vi "Vin_Vout_2015.vi"(2 "V in volt":dbl format="%0.2f", 3 "Fondo Scala 6024":dbl(ring)=10.0 items=["10"=10.0, "5"=5.0, "0.5"=0.5, "0.05"=0.05], 4 "Canale Ingresso":tag="Dev1/ai0", 5 "Canale uscita":tag="Dev1/ao0") -> (0 "standard deviation":dbl format="%.5f", 1 "mean Vout":dbl format="%.5f")   [LabVIEW 2014]
uses:
  <vilib>/DAQmx/write.llb/DAQmx Write (Analog DBL 1Chan 1Samp).vi
  <vilib>/DAQmx/read.llb/DAQmx Read (Analog 1D DBL 1Chan NSamp).vi
  <vilib>/DAQmx/create/channels.llb/DAQmx Create Channel (AO-Voltage-Basic).vi
  <vilib>/DAQmx/configure/timing.llb/DAQmx Timing (Sample Clock).vi
  <vilib>/DAQmx/miscellaneous.llb/DAQmx Fill In Error Info.vi
  <vilib>/DAQmx/create/channels.llb/DAQmx Create Channel (AI-Voltage-Basic).vi
  <vilib>/Analysis/NI_AALBase.lvlib
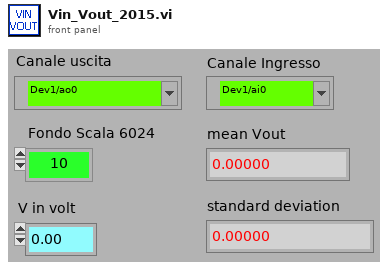
[diagram p1: front panel]
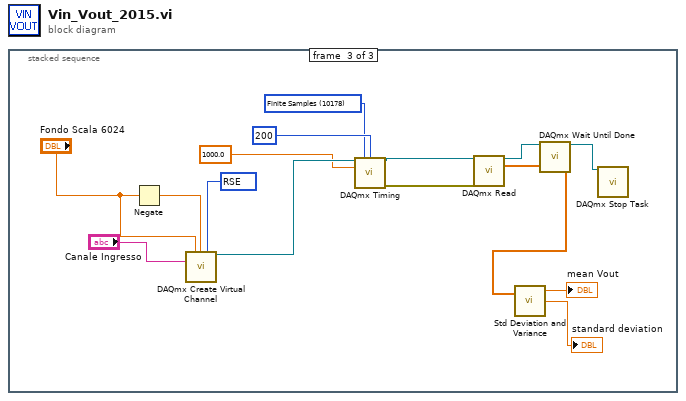
[diagram p0: block diagram]
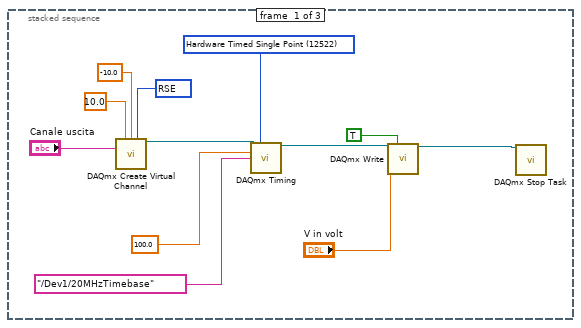
[diagram p2: hidden frame]
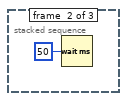
[diagram p3: hidden frame]
diagram:
  n1 = stacked-sequence {
    frame #0 {
      w7 = 12522 items=["Finite Samples"=10178, "Continuous Samples"=10123, "Hardware Timed Single Point"=12522] ("sample mode")
      w10 = 10083 items=["Default"=-1, "RSE"=10083, "Differential"=10106, "Pseudodifferential"=12529] ("output terminal configuration")
      n2 = call-poly <vilib>:"DAQmx Create Virtual Channel.vi"("maximum value"=10.0, "minimum value"=-10.0, "output terminal configuration"=w10, "physical channels"="Canale uscita") -> ("task out"=w9:refnum<k21>)  [unwired: 5 in, 6 out]
      n3 = call-poly <vilib>:"DAQmx Timing.vi"("task/channels in"=w9, "sample mode"=w7, "rate"=100.0, "source"=tag "/Dev1/20MHzTimebase") -> ("task out"=w6:refnum<k21>)  [unwired: 3 in, 8 out]
      n4 = call-poly <vilib>:"DAQmx Write.vi"("task/channels in"=w6, "auto start"=TRUE, "data"="V in volt") -> ("task out"=w4:refnum<k21>)  [unwired: 1 in, 11 out]
      n5 = call <vilib>:"DAQmx Stop Task.vi"("task/channels in"=w4) -> ()  [unwired: 1 in, 14 out]
    }
    frame #1 {
      n6 = Wait (ms)(milliseconds to wait=u32 50) -> ()  [unwired: 1 out]
    }
    frame #2 {
      w19 = 10178 items=["Finite Samples"=10178, "Continuous Samples"=10123, "Hardware Timed Single Point"=12522] ("sample mode")
      w27 = 10083 items=["default"=-1, "RSE"=10083, "NRSE"=10078, "Differential"=10106, "Pseudodifferential"=12529] ("input terminal configuration")
      n7 = Negate(x="Fondo Scala 6024") -> (-x=w28:dbl)
      n8 = call-poly <vilib>:"DAQmx Create Virtual Channel.vi"("maximum value"="Fondo Scala 6024", "minimum value"=w28, "input terminal configuration"=w27, "physical channels"="Canale Ingresso") -> ("task out"=w22:refnum<k21>)  [unwired: 5 in, 6 out]
      n9 = call-poly <vilib>:"DAQmx Timing.vi"("task/channels in"=w22, "sample mode"=w19, "samples per channel"=u32 200, "rate"=1000.0) -> ("task out"=w25:refnum<k21>, "error out"=w24:errorcluster)  [unwired: 3 in, 7 out]
      n10 = call-poly <vilib>:"DAQmx Read.vi"("task/channels in"=w25, "error in"=w24) -> ("task out"=w20:refnum<k21>, "data"=w17:dbl[])  [unwired: 1 in, 11 out]
      n11 = call <vilib>:"Std Deviation and Variance.vi"("X"=w17) -> ("mean"=→"mean Vout":dbl, "standard deviation"=→"standard deviation":dbl)  [unwired: 1 in, 1 out]
      n12 = call <vilib>:"DAQmx Wait Until Done.vi"("task/channels in"=w20) -> ("task out"=w18:refnum<k21>)  [unwired: 2 in, 12 out]
      n13 = call <vilib>:"DAQmx Stop Task.vi"("task/channels in"=w18) -> ()  [unwired: 1 in, 14 out]
    }
  }
